vi "PID elapsed time.vi"(7 "initialize":bool) -> (8 "elapsed time":dbl format="%.2f")   [LabVIEW 2016]
doc: "This one-shot returns the elapsed time since the previous call\n\nPaul K Dixon\nPhysics 350\nCSUSB Physics"
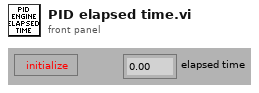
[diagram p1: front panel]
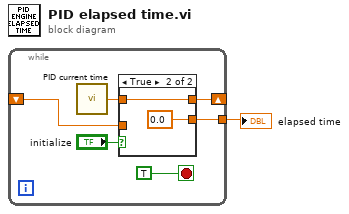
[diagram p0: block diagram]
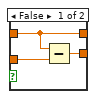
[diagram p2: hidden frame]
diagram:
  n1 = while {
    shift-left: _ -> [w4]
    shift-right: [w5] -> _
    tunnel: [w7] -> w1
    stop <- TRUE stop-if-true
    n2 = call "PID current time.vi"() -> ("current time (sec)"=w2:dbl)  [unwired: 15 in]
    n3 = case shown="True" "initialize" {
      tunnel: [w10 0.0 ("current time (sec)")] -> w7
      tunnel: [w8 w11] -> w5
      tunnel: w4 -> [w9 _]
      tunnel: w2 -> [w8 w11]
      frame False {
        n4 = Subtract(x=w8, y=w9) -> (x-y=w10:dbl)
      }
      frame True {
      }
    }
  }
  "elapsed time" <- w1
